vi "CALC_FILT_GATE_COUP_PAR_A.vi"(0 "VISA IN":refnum<visa-resource-name>, 1 "Parameters to Couple":i32, 5 "error in":errorcluster, 7 "Channel":i32) -> (14 "VISA Out":refnum<visa-resource-name>, 19 "error out":errorcluster)   [LabVIEW 2018, in "PNA-X.lvlib"]
doc: "CALCulate<cnum>:FILTer[:GATE]:COUPle:PARameters <num> \n(Read-Write) Specifies the time domain gating parameters to be coupled. The settings for those \nparameters will be copied from the selected measurement to all other measurements on the channel. \nTo enable Trace Coupling, use SENS:COUP:PAR \nTo specify Transform parameters to couple, use CALC:TRAN:COUP:PAR \nLearn more about Time Domain Trace Coupling \nSee Critical Note \nParameters \n<cnum> Channel number of the measurement. There must be a selected measurement \non that channel. If unspecified, <cnum> is set to 1. \n<num> (Numeric) Parameters to couple. To specify more than one parameter, add the \nnumbers. \n1 - Gating Stimulus (Start, Stop, Center, and Span TIME settings.) \n2 - Gating State (ON / OFF) \n4 - Gating Shape (Minimum, Normal, Wide, and Maximum) \n8 - Gating Type (Bandpass and Notch) \nExamples 'To couple all parameters: \nCALC:FILT:COUP:PAR 15 \n'To couple Stimulus and Type: \ncalculate2:filter:gate:couple:parameters 9 \nQuery Syntax CALCulate<cnum>:FILTer:GATE:COUPle:PARameters? \nReturn Type Numeric \nDefault 13 (All parameters except 2 - Gating State)"
uses:
  PNA-X.lvlib
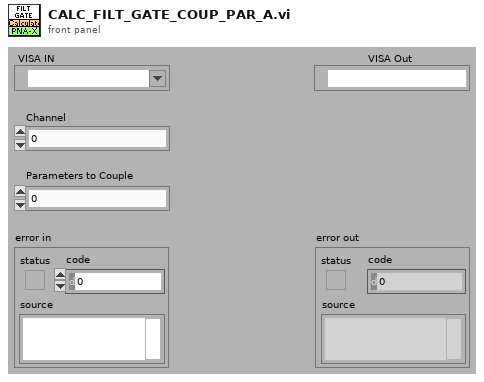
[diagram p1: front panel]
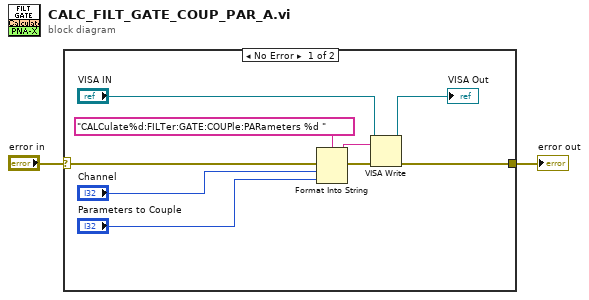
[diagram p0: block diagram]
diagram:
  n1 = case shown="No Error" "error in" {
    selector: "error in" -> [w11 w12]
    tunnel: [w6 w12] -> w1
    frame No Error {
      n2 = Format Into String(format string="CALCulate%d:FILTer:GATE:COUPle:PARameters %d " ("Cmdline"), error in=w11, "Channel", "Parameters to Couple") -> (resulting string=w9:string, error out=w10:errorcluster)  [unwired: 1 in]
      n3 = VISA Write(VISA resource name="VISA IN", write buffer=w9, error in (no error)=w10) -> (VISA resource name out=→"VISA Out":refnum<visa-resource-name>, error out=w6:errorcluster)  [unwired: 1 out]
    }
    frame Error {
    }
  }
  "error out" <- w1
